vi "readBinningXML.vi"(8 "error in (no error)":errorcluster, 10 "NativeXML in":refnum<class "NativeXML.lvclass">, 11 "PixelflySettings in":refnum<class "PixelflySettings.lvclass">) -> (0 "error out":errorcluster, 2 "NativeXML out":refnum<class "NativeXML.lvclass">, 3 "PixelflySettings out":refnum<class "PixelflySettings.lvclass">)   [LabVIEW 2009, in "Tools.lvlib" / "Settings.lvlib" / "PixelflySettings.lvclass"]
uses:
  PixelflySettings.lvclass
  NativeXML/NativeXML.lvclass
  PixelflySettings.lvclass/PixelflySettings.ctl
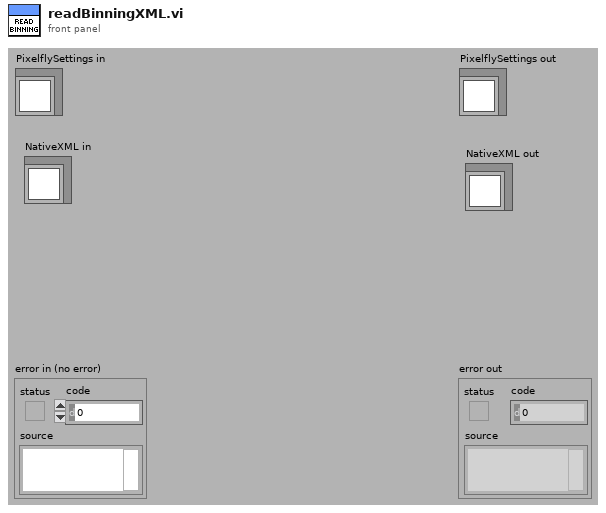
[diagram p1: front panel]
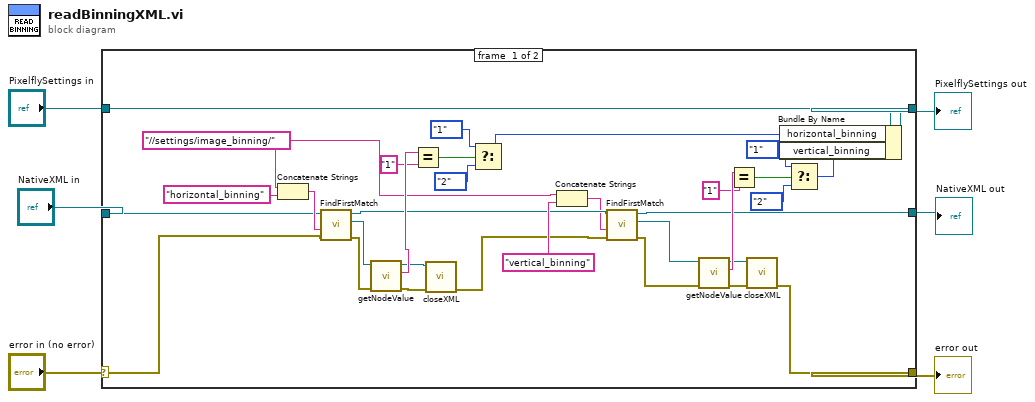
[diagram p0: block diagram]
diagram:
  n1 = case shown="No Error" "error in (no error)" {
    selector: "error in (no error)" -> [w15 w42]
    tunnel: [w21 w42] -> w5
    tunnel: [w26 w41] -> w3
    tunnel: "PixelflySettings in" -> [w27 w41]
    tunnel: "NativeXML in" -> [w13 w40]
    tunnel: [w12 w40] -> w1
    frame #0 {
      w19 = "//settings/image_binning/" ("searchElementIn")
      n2 = Concatenate Strings(w19, "horizontal_binning") -> (w14:string)
      n3 = call "FindFirstMatch.vi"("error in (no error)"=w15, "xPath"=w14, "NativeXML in"=w13) -> ("error out"=w17:errorcluster, "NativeXML match"=w16:refnum<class "NativeXML.lvclass">, "NativeXML out"=w11:refnum<class "NativeXML.lvclass">)  [unwired: 6 in]
      n4 = call "getNodeValue.vi"("error in (no error)"=w17, "NativeXML in"=w16) -> ("error out"=w24:errorcluster, "Value"=w39:string, "NativeXML out"=w25:refnum<class "NativeXML.lvclass">)  [unwired: 7 in]
      n5 = Equal?(x=w39, y="1") -> (x = y?=w37:bool)
      n6 = call "closeXML.vi"("error in (no error)"=w24, "NativeXML in"=w25) -> ("error out"=w10:errorcluster)  [unwired: 9 in]
      n7 = Select(t=enum16{"1", "2"}."1", s=w37, f=enum16{"1", "2"}."2") -> (s? t:f=w28:enum16{"1", "2"})
      n8 = Concatenate Strings(w19, "vertical_binning") -> (w7:string)
      n9 = call "FindFirstMatch.vi"("error in (no error)"=w10, "xPath"=w7, "NativeXML in"=w11) -> ("error out"=w9:errorcluster, "NativeXML match"=w8:refnum<class "NativeXML.lvclass">, "NativeXML out"=w12:refnum<class "NativeXML.lvclass">)  [unwired: 6 in]
      n10 = call "getNodeValue.vi"("error in (no error)"=w9, "NativeXML in"=w8) -> ("error out"=w22:errorcluster, "Value"=w34:string, "NativeXML out"=w23:refnum<class "NativeXML.lvclass">)  [unwired: 7 in]
      n11 = Equal?(x=w34, y="1") -> (x = y?=w32:bool)
      n12 = call "closeXML.vi"("error in (no error)"=w22, "NativeXML in"=w23) -> ("error out"=w21:errorcluster)  [unwired: 9 in]
      n13 = Select(t=enum16{"1", "2"}."1", s=w32, f=enum16{"1", "2"}."2") -> (s? t:f=w29:enum16{"1", "2"})
      n14 = Bundle By Name(cluster=w27, "horizontal_binning"=w28, "vertical_binning"=w29) -> (w26:refnum<class "PixelflySettings.lvclass">)
    }
    frame #1 {
    }
  }
  "error out" <- w5
  "PixelflySettings out" <- w3
  "NativeXML out" <- w1
